vi "Magazine_Globals.vi"() -> ()   [LabVIEW 2020]
uses:
  Subsystems/Arrow/Magazine_Cluster.ctl
  Subsystems/Arrow/Magazine_Control_States.ctl
panel:
  in  "Magazine_Motor_Value":dbl
  in  "Magazine_Execute_Notifier":refnum<notifier>
  in  "Magazine_Set_Notifier":refnum<notifier>
  in  "Magazine_Execute_Ref":string="Magazine_Execute_Ref"
  in  "Magazine_Set_Ref":string="Magazine_Set_Ref"
  in  "Magazine_Motor":string="Magazine_Motor"
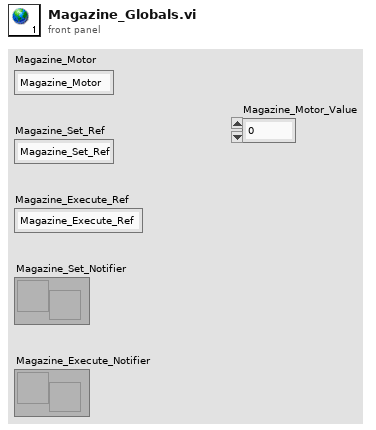
[diagram p1: front panel]
diagram:
